vi "Triggers-Stop.vi"(7 "Logging queue element":T1={"Imaging Protocol"=enum."Live Imaging", "Number of Trials"=0, "Frame Size"=512, "# Averaged frames"=0, "Dwell time (us)"=0.0, "Index of Z-plane"=0, "Timelapse?"=FALSE, "Logging process is active"=FALSE, "Speed logging enabled"=FALSE, "tdms file ref"=refnum, "path"=path "", "Trial Number"=0, "Expected # points acquired"=FALSE, "Manually stopped"=FALSE, "Last trial"=FALSE, "Ch0 data"=[], "Ch1 data"=[], "Ref Data"=[], "Ref Frame Time"=[], "Image Time"=[], "Continuous Time"=[], "Ref X Length"=0, "Ref Y Length"=0, "# Ref Averaged frames"=0, "Ref Dwell time (us)"=0.0, "Points acquired"={"Ch0 last trial"=0, "Ch1 last trial"=0, "All trials"=0}, "HW Timings File"=refnum} {"Ref Dwell time (us)" format="%#.6g"; "Frame Size" items=["100X100"=100, "128X128"=128, "200X200"=200, "256X256"=256, "512X512"=512, "1024x1024"=1024, "2048x2048"=2048]; "Dwell time (us)" format="%#.6g"}, 8 "error in (no error)":errorcluster, 11 "FPGA Ref":T5) -> (0 "error out":errorcluster)   [LabVIEW 2020]
uses:
  RIG-SPECIFIC FILES/FPGA Refs/FPGA Ref.ctl
  Typedefs/Logging queue element.ctl
  Typedefs/Imaging Protocols enum.ctl
  Typedefs/Frame Size.ctl
  Typedefs/Acquired points count.ctl
  Typedefs/Read Write Enum.ctl
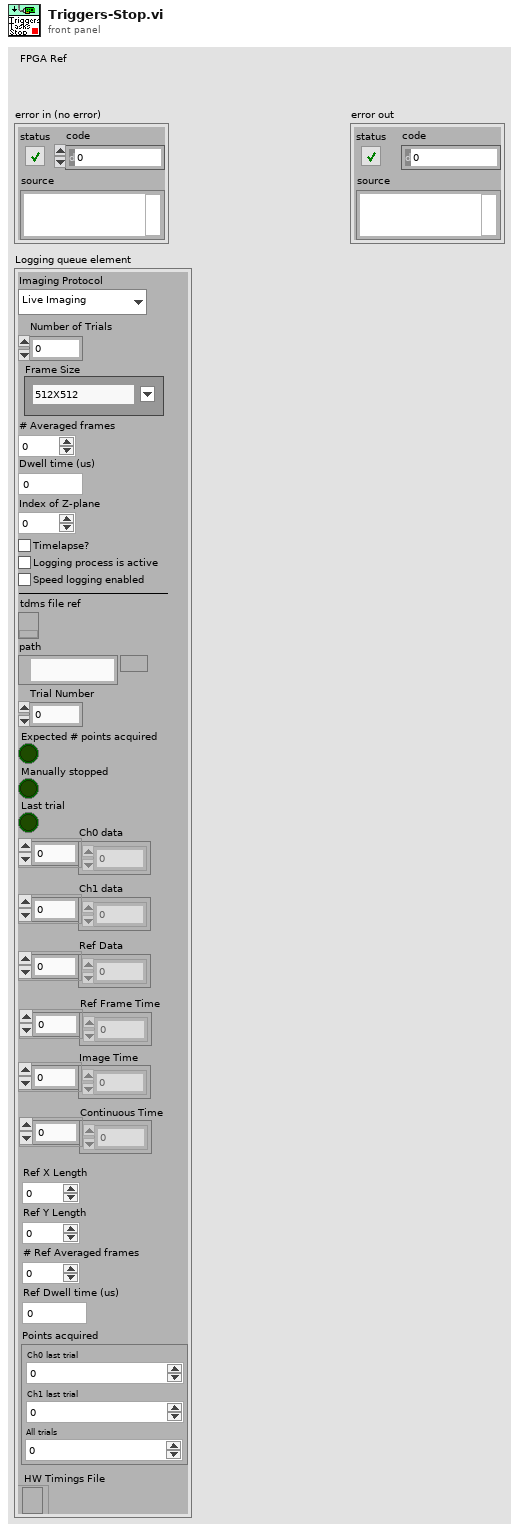
[diagram p1: front panel]
types:
  T1 = typedef "Logging queue element.ctl" = cluster{"Imaging Protocol":T2, "Number of Trials":u16, "Frame Size":T3, "# Averaged frames":u16, "Dwell time (us)":dbl, "Index of Z-plane":i32, "Timelapse?":bool, "Logging process is active":bool, "Speed logging enabled":bool, "tdms file ref":refnum<k34>, "path":path, "Trial Number":i32, "Expected # points acquired":bool, "Manually stopped":bool, "Last trial":bool, "Ch0 data":u32[], "Ch1 data":u32[], "Ref Data":u32[], "Ref Frame Time":u64[], "Image Time":u64[], "Continuous Time":u64[], "Ref X Length":u16, "Ref Y Length":u16, "# Ref Averaged frames":u16, "Ref Dwell time (us)":dbl, "Points acquired":T4, "HW Timings File":refnum<file>}
  T2 = typedef "Imaging Protocols enum.ctl" = enum16{"AOL Z-Stack", "Motor Z Stack", "Functional Acquisition", "Single Plane Acquisition", "Volume Acquisition", "Live Imaging", "Live Plane Imaging", "Live Volume Imaging"}
  T3 = typedef "Frame Size.ctl" = u16
  T4 = typedef "Acquired points count.ctl" = cluster{"Ch0 last trial":u64, "Ch1 last trial":u64, "All trials":u64}
  T5 = typedef "FPGA Ref.ctl" = refnum<k20>
  T6 = typedef "Read Write Enum.ctl" = enum16{"Read", "Write"}
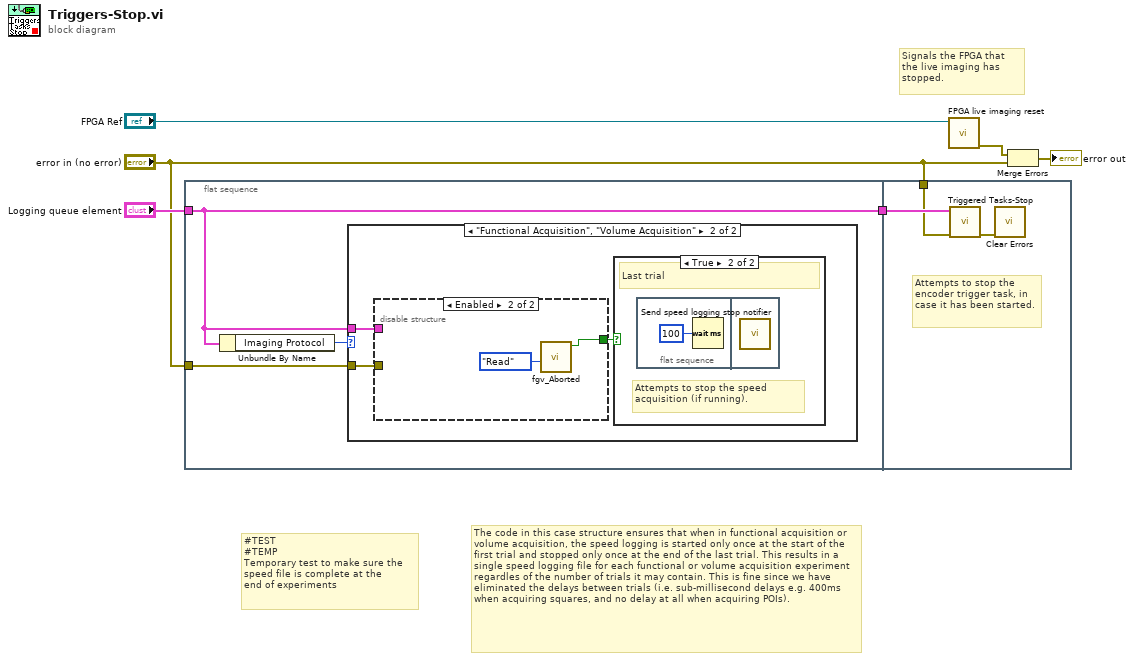
[diagram p0: block diagram]
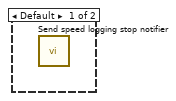
[diagram p2: hidden frame]
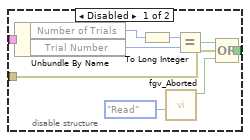
[diagram p3: hidden frame]
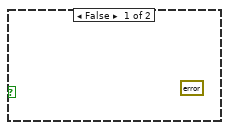
[diagram p4: hidden frame]
diagram:
  # "#TEST\n#TEMP\nTemporary test to make sure the \nspeed file is complete at the \nend of experiments"
  # "The code in this case structure ensures that when in functional acquisition or volume acquisition, the speed logging is started only once at the start of the first trial and stopped only once at the end of the last trial. This results in a single speed logging file for each functional or volume acquisition experiment regardles of the number of trials it may contain. This is fine since we have eliminated the delays between trials (i.e. sub-millisecond delays e.g. 400ms when acquiring squares, and no delay at all when acquiring POIs)."
  # "Signals the FPGA that the live imaging has stopped."
  n1 = flat-sequence {
    tunnel: "Logging queue element" -> [w7]
    tunnel: "error in (no error)" -> [w8]
    tunnel: [w7] -> w2
    tunnel: w2 -> [w26]
    tunnel: "error in (no error)" -> [w25]
    frame #0 {
      n2 = Unbundle By Name(w7) -> ("Imaging Protocol"=w9:T2)
      n3 = case shown="\"Functional Acquisition\", \"Volume Acquisition\"" w9 {
        tunnel: w7 -> [_ w12]
        tunnel: w8 -> [_ w10]
        frame Default {
          n4 = call "Send speed logging stop notifier.vi"() -> ()  [unwired: 11 in, 1 out]
        }
        frame "Functional Acquisition", "Volume Acquisition" {
          n5 = disable-structure shown="Enabled" {
            disable-tunnel: w12 -> [w18 _]
            disable-tunnel: [w15 w22] -> w11
            disable-tunnel: w10 -> [w14 _]
            frame Disabled {
              n6 = Unbundle By Name(w18) -> ("Number of Trials"=w20:u16, "Trial Number"=w21:i32)
              n7 = To Long Integer(number=w20) -> (32bit integer=w19:i32)
              n8 = call "fgv_Aborted.vi"("Function"=Read_Write_Enum."Read") -> ("Funct Acq Aborted?"=w13:bool)  [unwired: 9 in, 1 out]
              n9 = Equal?(x=w19, y=w21) -> (x = y?=w16:bool)
              n10 = Compound Arithmetic op=OR(w16, w14, w13) -> (w15:bool)
            }
            frame Enabled {
              n11 = call "fgv_Aborted.vi"("Function"=Read_Write_Enum."Read") -> ("Funct Acq Aborted?"=w22:bool)  [unwired: 9 in, 1 out]
            }
          }
          n12 = case shown="True" w11 {
            frame False {
              (unwired) errorcluster {"status"=FALSE, "code"=0, "source"=""} ("error out (No error)")
            }
            frame True {
              # "Attempts to stop the speed acquisition (if running)."
              # "Last trial"
              n13 = flat-sequence {
                frame #0 {
                  n14 = Wait (ms)(milliseconds to wait=u32 100) -> ()  [unwired: 1 out]
                }
                frame #1 {
                  n15 = call "Send speed logging stop notifier.vi"() -> ()  [unwired: 11 in, 1 out]
                }
              }
            }
          }
        }
      }
    }
    frame #1 {
      # "Attempts to stop the\nencoder trigger task, in \ncase it has been started."
      n16 = call "Triggered Tasks-Stop.vi"("error in (no error)"=w25, "Logging queue element"=w26) -> ("error out"=w27:errorcluster)  [unwired: 9 in]
      n17 = call <vilib>:"Clear Errors.vi"("error in (no error)"=w27) -> ()  [unwired: 5 in, 2 out]
    }
  }
  n18 = call "FPGA live imaging reset.vi"("FPGA VI Ref"="FPGA Ref") -> ("error out"=w5:errorcluster)  [unwired: 10 in]
  n19 = Merge Errors(w5, "error in (no error)") -> (→"error out":errorcluster)
